vi "GUID_Generator.vi"(8 "error in (no error)":errorcluster) -> (0 "error out":errorcluster, 3 "GUID String":string)   [LabVIEW 2013]
doc: "This VI generates a GUID which is an unique identifier used for standard EAS Databases."
panel:
  out "Numeric":i32
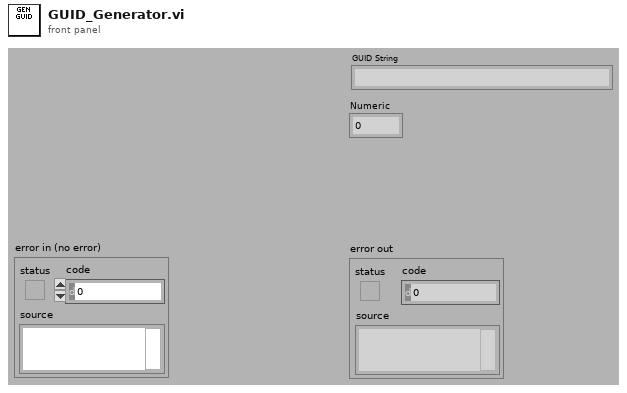
[diagram p1: front panel]
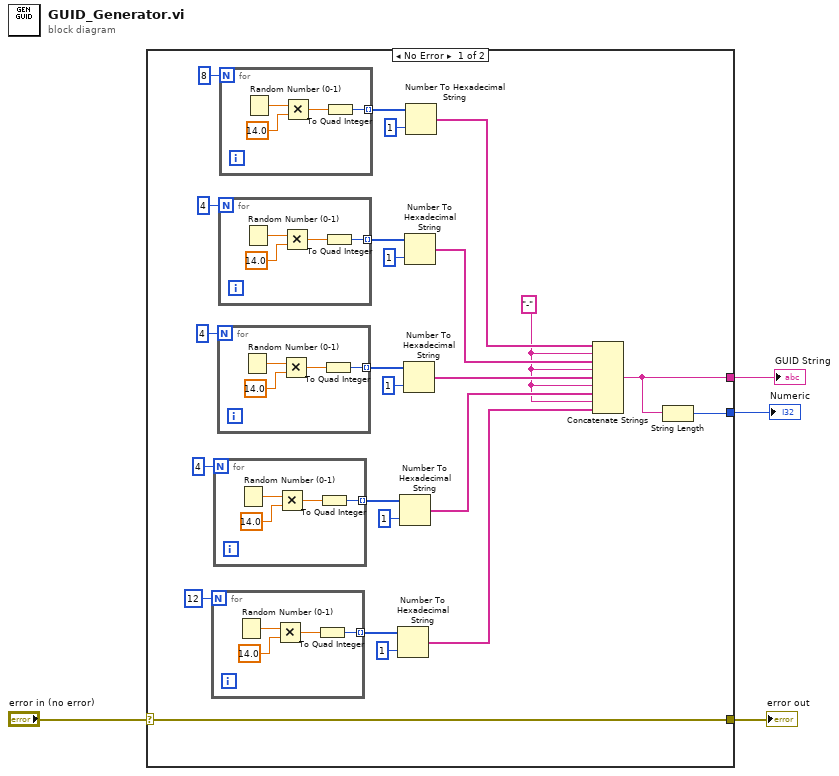
[diagram p0: block diagram]
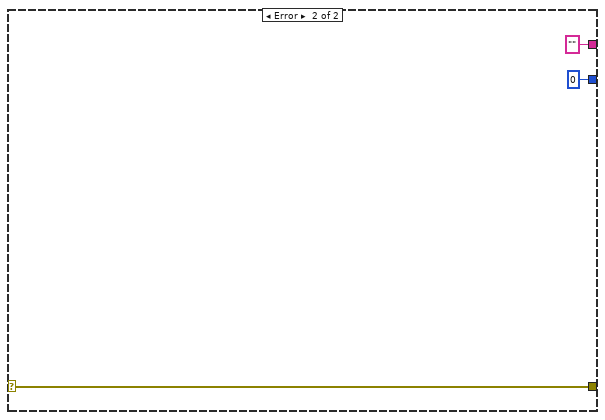
[diagram p2: hidden frame]
diagram:
  n1 = case shown="No Error" "error in (no error)" {
    selector: "error in (no error)" -> [w7 w51]
    tunnel: [w7 w51] -> w3
    tunnel: [w6 ""] -> w2
    tunnel: [w5 0] -> w1
    frame No Error {
      w8 = "-"
      n2 = for {
        N: 12 -> [_]
        tunnel: [w29] -> w15 mode=indexing
        n3 = Random Number (0-1)() -> (number: 0 to 1=w32:dbl)
        n4 = Multiply(x=w32, y=14.0) -> (x*y=w30:dbl)
        n5 = To Quad Integer(1:w30) -> (0:w29:i64)
      }
      n6 = for {
        N: 4 -> [_]
        tunnel: [w33] -> w18 mode=indexing
        n7 = Random Number (0-1)() -> (number: 0 to 1=w36:dbl)
        n8 = Multiply(x=w36, y=14.0) -> (x*y=w34:dbl)
        n9 = To Quad Integer(1:w34) -> (0:w33:i64)
      }
      n10 = for {
        N: 4 -> [_]
        tunnel: [w37] -> w21 mode=indexing
        n11 = Random Number (0-1)() -> (number: 0 to 1=w40:dbl)
        n12 = Multiply(x=w40, y=14.0) -> (x*y=w38:dbl)
        n13 = To Quad Integer(1:w38) -> (0:w37:i64)
      }
      n14 = for {
        N: 4 -> [_]
        tunnel: [w41] -> w24 mode=indexing
        n15 = Random Number (0-1)() -> (number: 0 to 1=w44:dbl)
        n16 = Multiply(x=w44, y=14.0) -> (x*y=w42:dbl)
        n17 = To Quad Integer(1:w42) -> (0:w41:i64)
      }
      n18 = for {
        N: 8 -> [_]
        tunnel: [w45] -> w27 mode=indexing
        n19 = Random Number (0-1)() -> (number: 0 to 1=w48:dbl)
        n20 = Multiply(x=w48, y=14.0) -> (x*y=w46:dbl)
        n21 = To Quad Integer(1:w46) -> (0:w45:i64)
      }
      n22 = Number To Hexadecimal String(1:i16 1 ("width (-)"), 2:w15) -> (0:w9:string[])
      n23 = Number To Hexadecimal String(1:i16 1 ("width (-)"), 2:w18) -> (0:w10:string[])
      n24 = Number To Hexadecimal String(1:i16 1 ("width (-)"), 2:w21) -> (0:w11:string[])
      n25 = Number To Hexadecimal String(1:i16 1 ("width (-)"), 2:w24) -> (0:w12:string[])
      n26 = Number To Hexadecimal String(1:i16 1 ("width (-)"), 2:w27) -> (0:w13:string[])
      n27 = Concatenate Strings(w13, w8, w12, w8, w11, w8, w10, w8, w9) -> (w6:string)
      n28 = String Length(string=w6) -> (length=w5:i32)
    }
    frame Error {
    }
  }
  "error out" <- w3
  "GUID String" <- w2
  "Numeric" <- w1
